vi "Scroll Multicolumn Listbox for New Selection.vi"(8 "error in":errorcluster, 10 "new index":i32, 11 "MulticolumnListbox":refnum<vi>) -> (0 "error out":errorcluster)   [LabVIEW 2018, in "NI_TDMS File Viewer.lvlib"]
uses:
  NI_TDMS File Viewer.lvlib
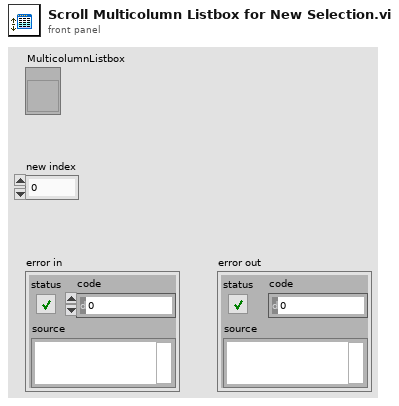
[diagram p1: front panel]
types:
  T1 = typedef "LVRowAndColumnUnsignedTypeDef.ctl" = cluster{"Row":u32, "Column":u32}
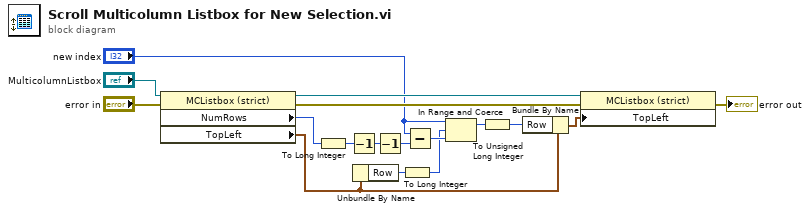
[diagram p0: block diagram]
diagram:
  n1 = property on="Property Node" class="MCListbox (strict)"(reference="MulticolumnListbox", error in="error in") -> (reference out=w8:refnum<vi>, error out=w16:errorcluster, "NumRows"=w11:u32, "TopLeft"=w10:T1)
  n2 = To Long Integer(number=w11) -> (32bit integer=w4:i32)
  n3 = Decrement(x=w4) -> (x-1=w13:i32)
  n4 = Unbundle By Name(w10) -> ("Row"=w7:u32)
  n5 = Decrement(x=w13) -> (x-1=w14:i32)
  n6 = To Long Integer(number=w7) -> (32bit integer=w3:i32)
  n7 = Subtract(x="new index", y=w14) -> (x-y=w6:i32)
  n8 = In Range and Coerce(upper limit="new index", x=w3, lower limit=w6) -> (coerced(x)=w5:i32)  [unwired: 1 out]
  n9 = To Unsigned Long Integer(number=w5) -> (unsigned 32bit integer=w2:u32)
  n10 = Bundle By Name(cluster=w10, "Row"=w2) -> (w12:T1)
  n11 = property on="Property Node" class="MCListbox (strict)"(reference=w8, error in=w16, "TopLeft"=w12) -> (error out=→"error out":errorcluster)  [unwired: 1 out]
